vi "Mail Post Sub Steps.vi"(10 "Mail Out":T1={"Configure Server"={"Outgoing Mail Server (SMTP)"="smtp.gmail.com", "Port"="587", "Sender's Email Address"="ltt24012025@gmail.com", "username"="ltt24012025@gmail.com", "password"="hhib mwaf mimz fohz", "Enable TLS"=TRUE}, "Data"={"Subject"="", "Message"="", "TO"=[], "CC"=[]}, "Sent"=FALSE, "MAIL Operation"=enum."Init"}, 11 "Sequence Context In":refnum<k7>) -> (0 "error out":errorcluster, 3 "Report Text":string)   [LabVIEW 2023, in "LTT_TeststandSteptypes.lvlib"]
uses:
  LTT_TeststandSteptypes.lvlib
  Control/Mail Data.ctl
  Control/Configure Mail Setting.ctl
  Control/Mail Message Data.ctl
  HardwareAbstractionLayer_LVOOP/Mail/Mail.lvclass
  HardwareAbstractionLayer_LVOOP/Database/Database.lvclass
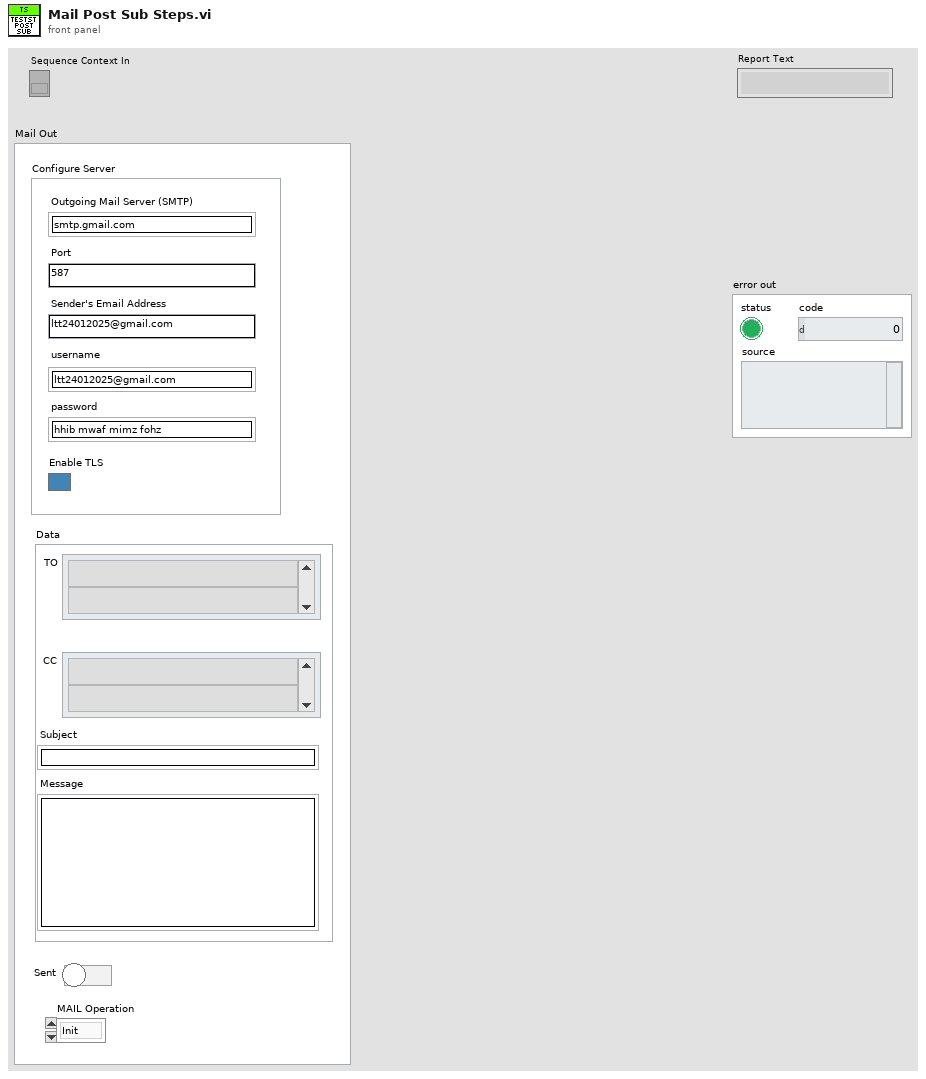
[diagram p1: front panel]
types:
  T1 = typedef "LTT_TeststandSteptypes.lvlib/Mail Data.ctl" = cluster{"Configure Server":T2, "Data":T3, "Sent":bool, "MAIL Operation":enum32{"Init", "Configure", "Sent", "Close"}}
  T2 = typedef "LTT_TeststandSteptypes.lvlib/Configure Mail Setting.ctl" = cluster{"Outgoing Mail Server (SMTP)":string, "Port":string, "Sender's Email Address":string, "username":string, "password":string, "Enable TLS":bool}
  T3 = typedef "LTT_TeststandSteptypes.lvlib/Mail Message Data.ctl" = cluster{"Subject":string, "Message":string, "TO":string[], "CC":string[]}
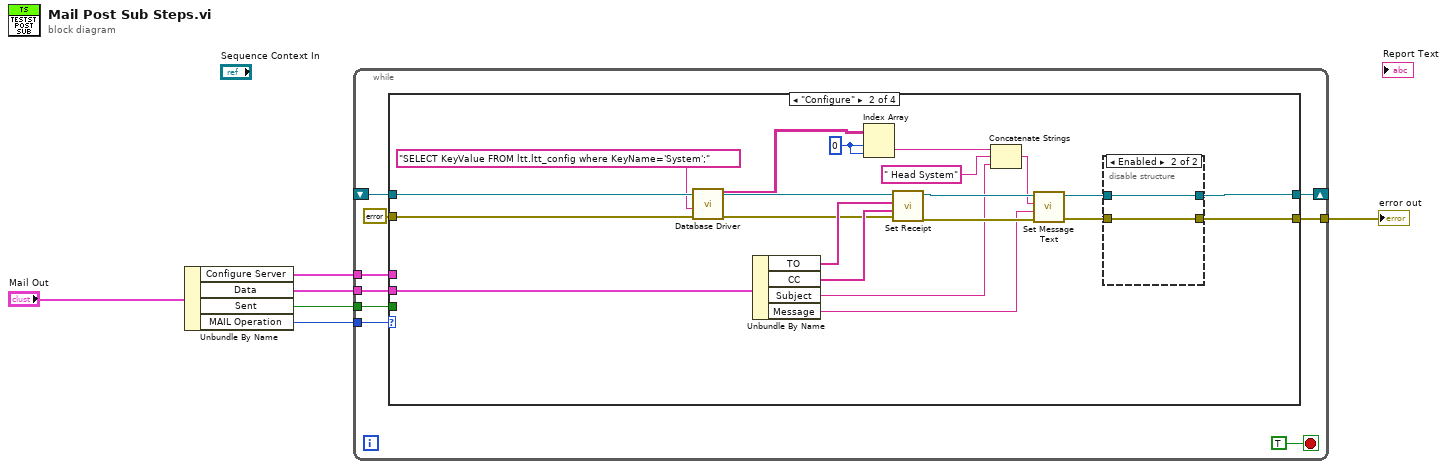
[diagram p0: block diagram]
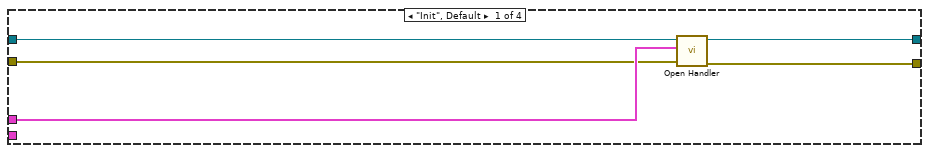
[diagram p2: hidden frame]
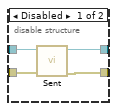
[diagram p3: hidden frame]
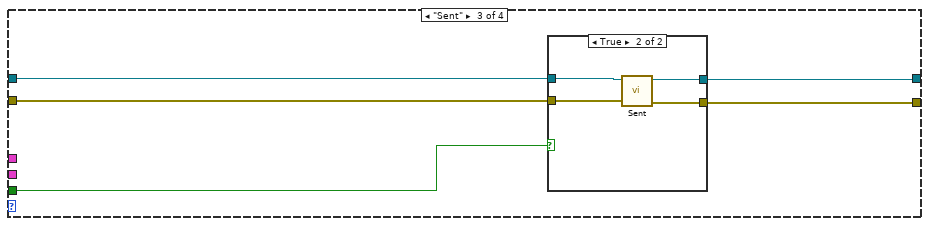
[diagram p4: hidden frame]
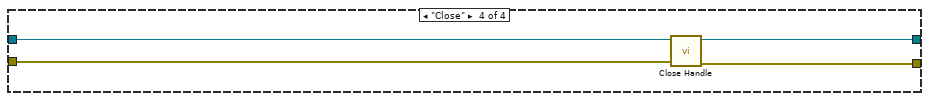
[diagram p6: hidden frame]
diagram:
  n1 = Unbundle By Name("Mail Out") -> ("Configure Server"=w4:T2, "Data"=w2:T3, "Sent"=w1:bool, "MAIL Operation"=w5:enum32{"Init", "Configure", "Sent", "Close"})
  n2 = while {
    tunnel: w5 -> [w14]
    shift-right: [w12] -> _
    shift-left: _ -> [w13]
    tunnel: w4 -> [w11]
    tunnel: [w10] -> w3
    tunnel: w2 -> [w9]
    tunnel: w1 -> [w7]
    stop <- TRUE stop-if-true
    n3 = case shown="\"Configure\"" w14 {
      tunnel: w13 -> [w20 w40 w51 w61]
      tunnel: [w19 w22 w50 w60] -> w12
      tunnel: w11 -> [w18 _ _ _]
      tunnel: [w17 w21 w49 w59] -> w10
      tunnel: w9 -> [_ w37 _ _]
      tunnel: errorcluster {"status"=FALSE, "code"=0, "source"=""} ("error in (no error)") -> [w16 w26 w48 w58]
      tunnel: w7 -> [_ _ w47 _]
      frame "Init", Default {
        n4 = call-dynamic "Open Handler.vi"("error in (no error)"=w16, "Configure Server"=w18, "Mail in"=w20) -> ("error out"=w17:errorcluster, "Mail out"=w19:refnum<class "Mail.lvclass">)  [unwired: 7 in]
      }
      frame "Configure" {
        w32 = 0 ("index (row)")
        n5 = call "Database Driver.vi"("error in"=w26, "SQL query"="SELECT KeyValue FROM ltt.ltt_config where KeyName='System';") -> ("error out"=w25:errorcluster, "data"=w33:string[][])  [unwired: 6 in, 2 out]
        n6 = Unbundle By Name(w37) -> ("TO"=w36:string[], "CC"=w35:string[], "Subject"=w27:string, "Message"=w34:string)
        n7 = Index Array(array=w33, index (row)=w32, index (col)=w32) -> (element=w30:string)
        n8 = call-dynamic "Set Receipt.vi"("error in (no error)"=w25, "CC"=w35, "TO"=w36, "Mail in"=w40) -> ("error out"=w38:errorcluster, "Mail out"=w39:refnum<class "Mail.lvclass">)  [unwired: 6 in]
        n9 = Concatenate Strings(w30, " Head System" ("string"), w27) -> (w28:string)
        n10 = call-dynamic "Set Message Text.vi"("error in (no error)"=w38, "Message"=w34, "Subject"=w28, "Mail in"=w39) -> ("error out"=w23:errorcluster, "Mail out"=w24:refnum<class "Mail.lvclass">)  [unwired: 6 in]
        n11 = disable-structure shown="Enabled" {
          disable-tunnel: w24 -> [w44 w45]
          disable-tunnel: w23 -> [w43 w46]
          disable-tunnel: [w42 w45] -> w22
          disable-tunnel: [w41 w46] -> w21
          frame Disabled {
            n12 = call-dynamic "Sent.vi"("error in (no error)"=w43, "Mail in"=w44) -> ("error out"=w41:errorcluster, "Mail out"=w42:refnum<class "Mail.lvclass">)  [unwired: 8 in]
          }
          frame Enabled {
          }
        }
      }
      frame "Sent" {
        n13 = case shown="True" w47 {
          tunnel: w51 -> [w53 w57]
          tunnel: [w53 w56] -> w50
          tunnel: [w52 w55] -> w49
          tunnel: w48 -> [w52 w54]
          frame False {
          }
          frame True {
            n14 = call-dynamic "Sent.vi"("error in (no error)"=w54, "Mail in"=w57) -> ("error out"=w55:errorcluster, "Mail out"=w56:refnum<class "Mail.lvclass">)  [unwired: 8 in]
          }
        }
      }
      frame "Close" {
        n15 = call-dynamic "Close Handle.vi"("error in (no error)"=w58, "Mail in"=w61) -> ("error out"=w59:errorcluster, "Mail out"=w60:refnum<class "Mail.lvclass">)  [unwired: 8 in]
      }
    }
  }
  "error out" <- w3
